vi "Ejercicio_16_Histerisis.vi"() -> ()   [LabVIEW 2020]
panel:
  in  "?":bool
  out "Actuador":bool
  in  "Temperatura":dbl
  # "Simulación"
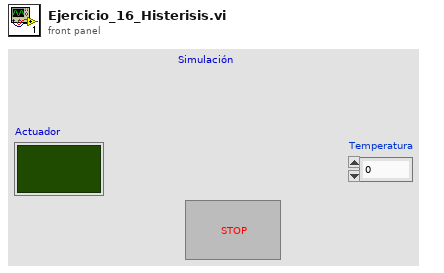
[diagram p1: front panel]
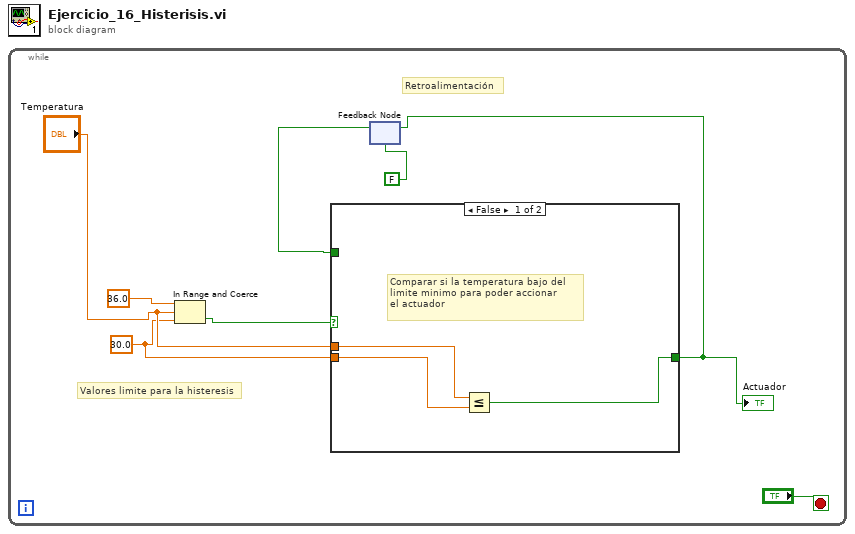
[diagram p0: block diagram]
diagram:
  n1 = while {
    stop <- "?" stop-if-true
    w5 = 30.0 ("lower limit")
    # "Retroalimentación"
    # "Valores limite para la histeresis"
    n2 = In Range and Coerce(upper limit=36.0, x="Temperatura", lower limit=w5) -> (In Range?=w7:bool)  [unwired: 1 out]
    n3 = feedback #1(FALSE) -> (w2:bool)
    n4 = case shown="False" w7 {
      tunnel: "Temperatura" -> [w11 _]
      tunnel: w5 -> [w10 _]
      tunnel: [w9 w12] -> w4
      tunnel: w2 -> [_ w12]
      frame False {
        # "Comparar si la temperatura bajo del \nlimite minimo para poder accionar \nel actuador"
        n5 = Less Or Equal?(x=w11, y=w10) -> (x <= y?=w9:bool)
      }
      frame True {
      }
    }
    "Actuador" <- w4
    n6 = feedback-in #1(w4) -> ()
  }
